vi "Test Serialize.vi"(8 "error in (no error)":errorcluster) -> (0 "error out":errorcluster)   [LabVIEW 2013]
uses:
  <vilib>/addons/_JKI Toolkits/Caraya/classes/Test/Test.lvclass
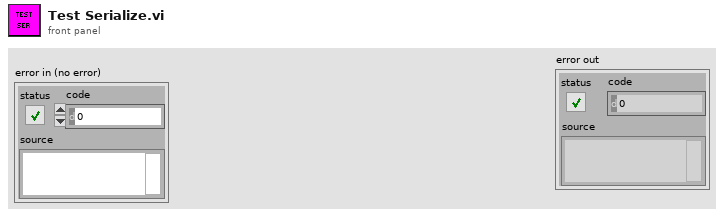
[diagram p1: front panel]
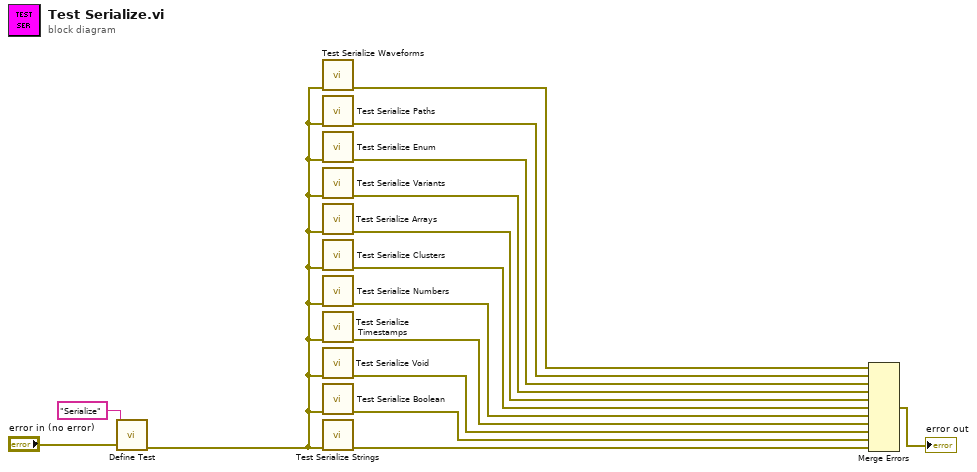
[diagram p0: block diagram]
diagram:
  n1 = call <vilib>:"Define Test.vi"("error in (no error)"="error in (no error)", "Label (VI Title)"="Serialize") -> ("error out"=w2:errorcluster)  [unwired: 9 in]
  n2 = call "Test Serialize Waveforms.vi"("error in (no error)"=w2) -> ("error out"=w1:errorcluster)  [unwired: 10 in]
  n3 = call "Test Serialize Paths.vi"("error in (no error)"=w2) -> ("error out"=w3:errorcluster)  [unwired: 10 in]
  n4 = call "Test Serialize Enum.vi"("error in (no error)"=w2) -> ("error out"=w4:errorcluster)  [unwired: 10 in]
  n5 = call "Test Serialize Variants.vi"("error in (no error)"=w2) -> ("error out"=w5:errorcluster)  [unwired: 10 in]
  n6 = call "Test Serialize Arrays.vi"("error in (no error)"=w2) -> ("error out"=w12:errorcluster)  [unwired: 10 in]
  n7 = call "Test Serialize Clusters.vi"("error in (no error)"=w2) -> ("error out"=w11:errorcluster)  [unwired: 10 in]
  n8 = call "Test Serialize Numbers.vi"("error in (no error)"=w2) -> ("error out"=w10:errorcluster)  [unwired: 10 in]
  n9 = call "Test Serialize Timestamps.vi"("error in (no error)"=w2) -> ("error out"=w9:errorcluster)  [unwired: 10 in]
  n10 = call "Test Serialize Void.vi"("error in (no error)"=w2) -> ("error out"=w8:errorcluster)  [unwired: 10 in]
  n11 = call "Test Serialize Boolean.vi"("error in (no error)"=w2) -> ("error out"=w7:errorcluster)  [unwired: 10 in]
  n12 = call "Test Serialize Strings.vi"("error in (no error)"=w2) -> ("error out"=w6:errorcluster)  [unwired: 10 in]
  n13 = Merge Errors(w1, w3, w4, w5, w12, w11, w10, w9, w8, w7, w6) -> (→"error out":errorcluster)
